vi "DSF.Shared.Configuration.Transfer.New.vi"(8 "error in (no error)":errorcluster, 10 "name":string, 11 "Transfer Configuration type":refnum<class "DSF.Shared.Configuration.Transfer.lvclass">) -> (0 "error out":errorcluster, 3 "Transfer Configuration out":refnum<class "DSF.Shared.Configuration.Transfer.lvclass">)   [LabVIEW 2016, in "DSF.Shared.lvlib" / "DSF.Shared.Configuration.Transfer.lvclass"]
uses:
  DSF.Shared.Configuration.Transfer.lvclass
  C:/Git/Sourcetree/DSF/Source/Shared/Classes/Configuration/DSF.Shared.Configuration.lvclass
  Channel/DSF.Shared.Configuration.Channel Array.lvclass
  DSF.Shared.Configuration.Transfer.lvclass/DSF.Shared.Configuration.Transfer.ctl
  Typedefs/DSF.Shared.Typedefs.Byte Order.ctl
  Configuration/DSF.Shared.Configuration.lvclass
  DSF.Shared.lvlib
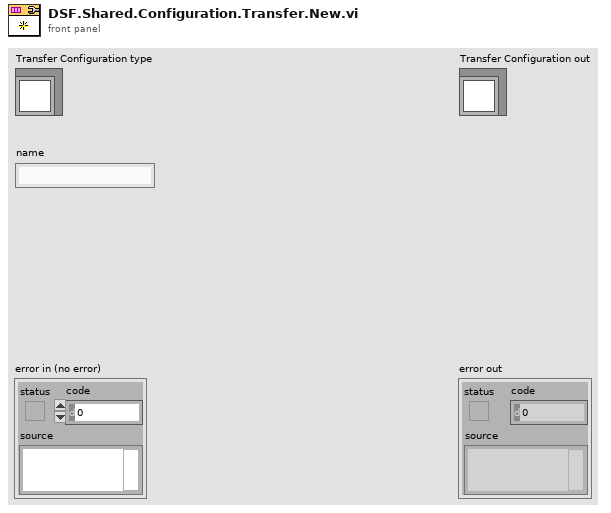
[diagram p1: front panel]
types:
  T1 = typedef "DSF.Shared.lvlib/DSF.Shared.Typedefs.Byte Order.ctl" = enum8{"big-endian", "little-endian"}
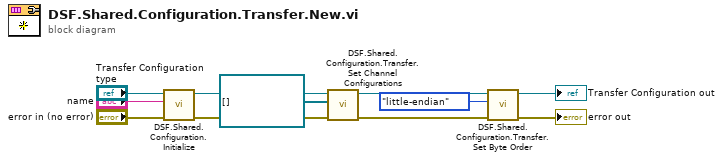
[diagram p0: block diagram]
diagram:
  n1 = call "DSF.Shared.Configuration.Initialize.vi"("error in (no error)"="error in (no error)", "name"="name", "Configuration in"="Transfer Configuration type") -> ("error out"=→"error out":errorcluster, "Configuration out"=w4:refnum<class "DSF.Shared.Configuration.Transfer.lvclass">)  [unwired: 7 in]
  n2 = call "DSF.Shared.Configuration.Transfer.Set Channel Configurations.vi"("Channel Configurations"=refnum<class "DSF.Shared.Configuration.Channel Array.lvclass">[] [], "Transfer Configuration in"=w4) -> ("Transfer Configuration out"=w9:refnum<class "DSF.Shared.Configuration.Transfer.lvclass">)  [unwired: 9 in]
  n3 = call "DSF.Shared.Configuration.Transfer.Set Byte Order.vi"("byte order"=DSF.Shared.Typedefs.Byte_Order."little-endian", "Transfer Configuration in"=w9) -> ("Transfer Configuration out"=→"Transfer Configuration out":refnum<class "DSF.Shared.Configuration.Transfer.lvclass">)  [unwired: 9 in]
